vi "G#Debugger_ProxyCall.vi"(0 "Method":i32, 1 "ObjectID":u32, 2 "ObjectAttributes (T)":bool=TRUE, 4 "Text":string, 5 "error in (no error)":errorcluster) -> (15 "Attributes":variant[](array[variant]), 16 "AllObjects":T1(array[cluster]), 17 "ObjectIDs":u32[](array[numeric]), 18 "ValidObject":bool, 19 "error out":errorcluster)   [LabVIEW 2020, in "G#Debugger.lvlib"]
uses:
  <vilib>/addons/_AddQ/G#Debugger/G#Debugger.lvlib
  <vilib>/addons/_AddQ/G#Object/G#Object.lvclass
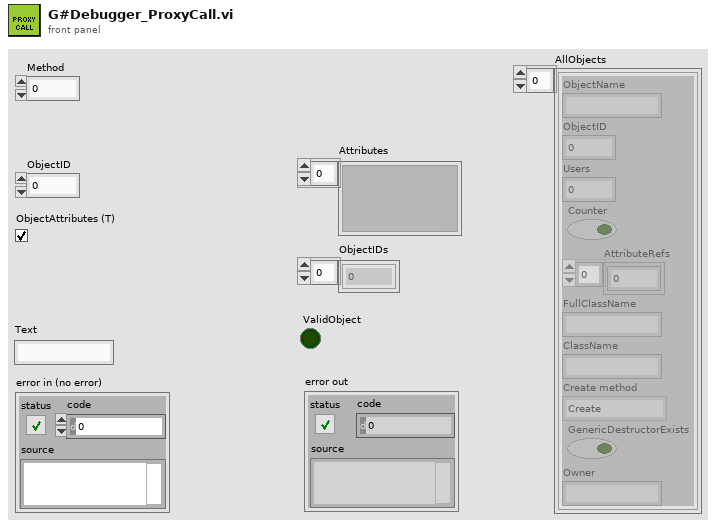
[diagram p1: front panel]
types:
  T1 = cluster{"ObjectName":string, "ObjectID":u32, "Users":i32, "Counter":bool, "AttributeRefs":u32[], "FullClassName":string, "ClassName":string, "Create method":enum16{"Create", "Create or look up existing", "Look up existing"}, "GenericDestructorExists":bool, "Owner":string}[]
  T2 = typedef "G#Object.lvclass/G#Object_ObjectInfoType.ctl" = cluster{"ObjectName":string, "ObjectID":u32, "Users":i32, "Counter":bool, "AttributeRefs":u32[], "FullClassName":string, "ClassName":string, "CreateMethod":T3, "GenericDestructorExists":bool, "Owner":string}
  T3 = typedef "G#Object.lvclass/G#Object_CreateMethod.ctl" = enum16{"Create", "Create or look up existing", "Look up existing"}
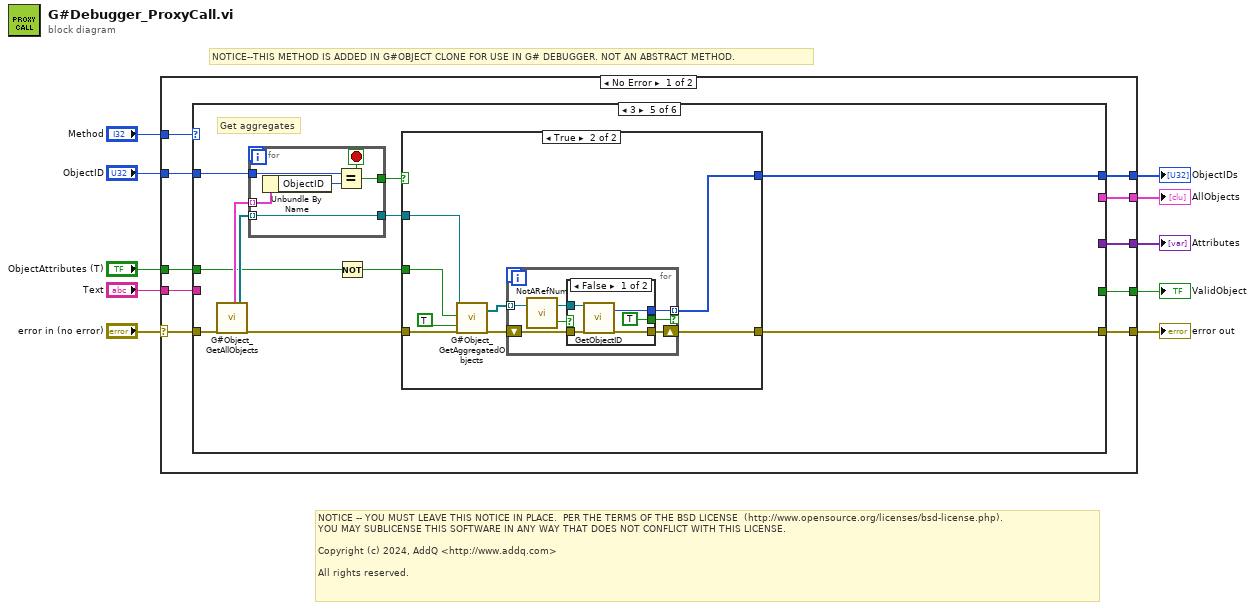
[diagram p0: block diagram]
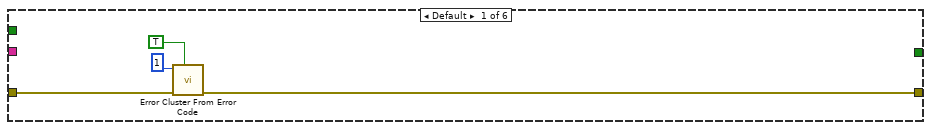
[diagram p2: hidden frame]
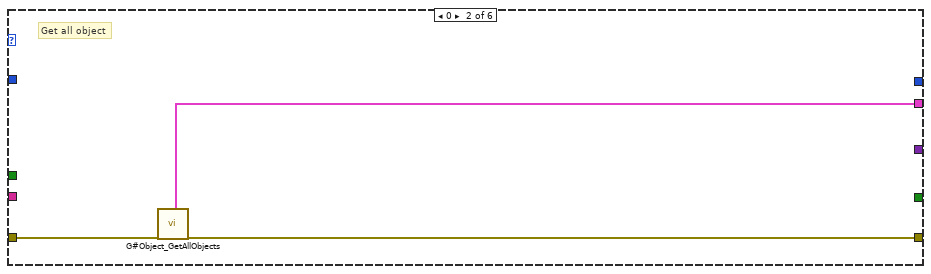
[diagram p3: hidden frame]
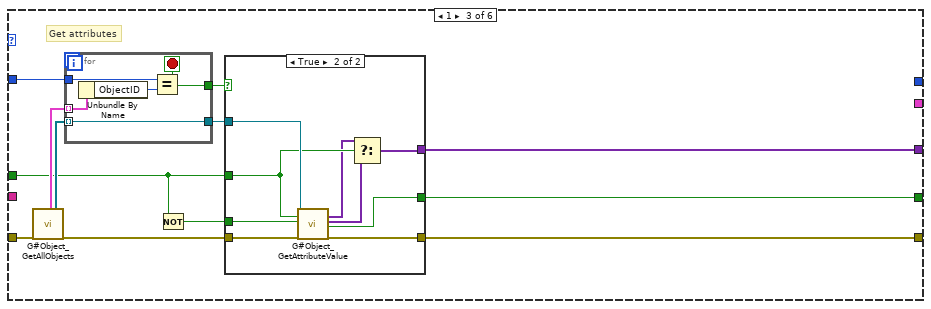
[diagram p4: hidden frame]
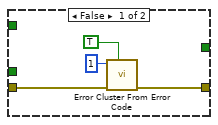
[diagram p5: hidden frame]
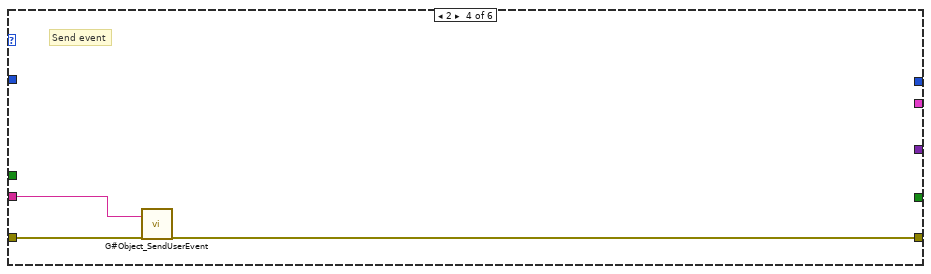
[diagram p6: hidden frame]
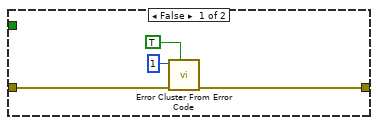
[diagram p7: hidden frame]
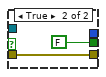
[diagram p8: hidden frame]
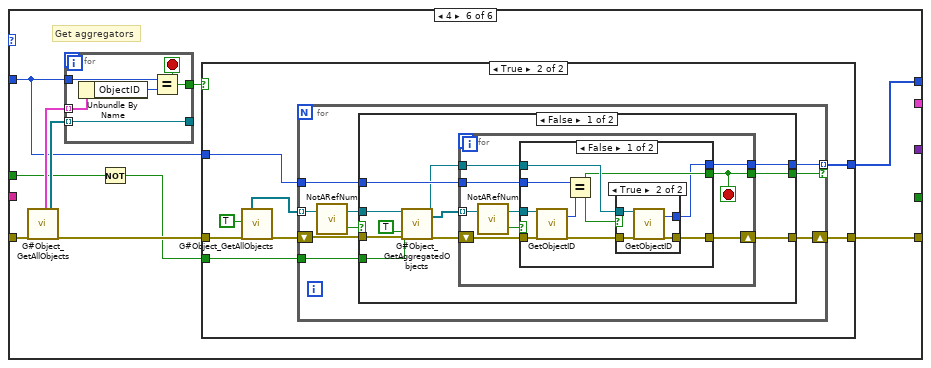
[diagram p9: hidden frame]
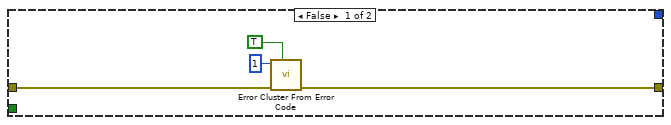
[diagram p10: hidden frame]
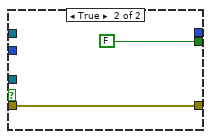
[diagram p12: hidden frame]
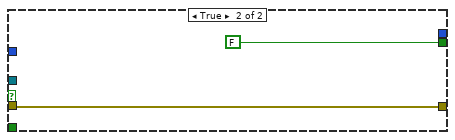
[diagram p13: hidden frame]
diagram:
  # "NOTICE--THIS METHOD IS ADDED IN G#OBJECT CLONE FOR USE IN G# DEBUGGER. NOT AN ABSTRACT METHOD."
  # "NOTICE -- YOU MUST LEAVE THIS NOTICE IN PLACE.  PER THE TERMS OF THE BSD LICENSE  (http://www.opensource.org/licenses/bsd-license.php).\nYOU MAY SUBLICENSE THIS SOFTWARE IN ANY WAY THAT DOES NOT CONFLICT WITH THIS LICENSE.\n\nCopyright (c) 2024, AddQ <http://www.addq.com>\n\nAll rights reserved."
  n1 = case shown="No Error" "error in (no error)" {
    selector: "error in (no error)" -> [w17 w177]
    tunnel: "ObjectID" -> [w20 _]
    tunnel: "ObjectAttributes (T)" -> [w16 _]
    tunnel: [w19 w177] -> w8
    tunnel: [w15 _] -> w7
    tunnel: [w18 _] -> w6
    tunnel: "Method" -> [w14 _]
    tunnel: [w13 _] -> w3
    tunnel: "Text" -> [w12 _]
    tunnel: [w11 _] -> w1
    frame No Error {
      n2 = case shown="3" w14 {
        tunnel: w20 -> [_ _ w38 _ w70 w106]
        tunnel: [w21 w26 w34 w59 w62 w103] -> w19
        tunnel: [_ _ w33 _ _ _] -> w18
        tunnel: w17 -> [w23 w27 w32 w60 w68 w110]
        tunnel: w16 -> [_ _ w30 _ w67 w109]
        tunnel: [_ _ w29 _ _ _] -> w15
        tunnel: [_ w25 _ _ _ _] -> w13
        tunnel: w12 -> [_ _ _ w58 _ _]
        tunnel: [_ _ _ _ w63 w104] -> w11
        frame Default {
          n3 = call <vilib>:"Error Cluster From Error Code.vi"("show call chain? (False)"=TRUE, "error in (no error)"=w23, "error code (0)"=1) -> ("error out"=w21:errorcluster)  [unwired: 6 in]
        }
        frame 0 {
          # "Get all object"
          n4 = call <vilib>:"G#Object_GetAllObjects.vi"("error in (no error)"=w27) -> ("all objects"=w25:T2[], "error out"=w26:errorcluster)  [unwired: 15 in, 2 out]
        }
        frame 1 {
          # "Get attributes"
          n5 = call <vilib>:"G#Object_GetAllObjects.vi"("error in (no error)"=w32) -> ("all objects"=w39:T2[], "all refs"=w37:refnum<class "G#Object.lvclass">[], "error out"=w35:errorcluster)  [unwired: 15 in, 1 out]
          n6 = for {
            tunnel: w39 -> [w55] mode=indexing
            tunnel: w38 -> [w57]
            tunnel: w37 -> [w54] mode=indexing
            tunnel: [w54] -> w36
            tunnel: [w53] -> w28
            stop <- w53 stop-if-true
            n7 = Unbundle By Name(w55) -> ("ObjectID"=w56:u32)
            n8 = Equal?(x=w57, y=w56) -> (x = y?=w53:bool)
          }
          n9 = Not(x=w30) -> (.not. x?=w31:bool)
          n10 = case shown="True" w28 {
            tunnel: w36 -> [_ w52]
            tunnel: w35 -> [w41 w51]
            tunnel: [w40 w50] -> w34
            tunnel: [_ w49] -> w33
            tunnel: w31 -> [_ w48]
            tunnel: w30 -> [_ w47]
            tunnel: [_ w44] -> w29
            frame False {
              n11 = call <vilib>:"Error Cluster From Error Code.vi"("show call chain? (False)"=TRUE, "error in (no error)"=w41, "error code (0)"=1) -> ("error out"=w40:errorcluster)  [unwired: 6 in]
            }
            frame True {
              n12 = call <vilib>:"G#Object_GetAttributeValue.vi"("reference in"=w52, "object attributes (T)"=w47, "class attributes (F)"=w48, "error in (no error)"=w51) -> ("attributes"=w45:variant[], "class attributes"=w46:variant[], "valid object"=w49:bool, "error out"=w50:errorcluster)  [unwired: 11 in, 1 out]
              n13 = Select(t=w45, s=w47, f=w46) -> (s? t:f=w44:variant[])
            }
          }
        }
        frame 2 {
          # "Send event"
          n14 = call <vilib>:"G#Object_SendUserEvent.vi"("text"=w58, "error in (no error)"=w60) -> ("error out"=w59:errorcluster)  [unwired: 16 in, 1 out]
        }
        frame 3 {
          # "Get aggregates"
          n15 = call <vilib>:"G#Object_GetAllObjects.vi"("error in (no error)"=w68) -> ("all objects"=w71:T2[], "all refs"=w69:refnum<class "G#Object.lvclass">[], "error out"=w64:errorcluster)  [unwired: 15 in, 1 out]
          n16 = for {
            tunnel: w71 -> [w100] mode=indexing
            tunnel: w70 -> [w102]
            tunnel: w69 -> [w99] mode=indexing
            tunnel: [w99] -> w66
            tunnel: [w98] -> w61
            stop <- w98 stop-if-true
            n17 = Unbundle By Name(w100) -> ("ObjectID"=w101:u32)
            n18 = Equal?(x=w102, y=w101) -> (x = y?=w98:bool)
          }
          n19 = Not(x=w67) -> (.not. x?=w65:bool)
          n20 = case shown="True" w61 {
            tunnel: w66 -> [_ w81]
            tunnel: w65 -> [_ w80]
            tunnel: w64 -> [w73 w79]
            tunnel: [_ w78] -> w63
            tunnel: [w72 w77] -> w62
            frame False {
              n21 = call <vilib>:"Error Cluster From Error Code.vi"("show call chain? (False)"=TRUE, "error in (no error)"=w73, "error code (0)"=1) -> ("error out"=w72:errorcluster)  [unwired: 6 in]
            }
            frame True {
              n22 = call <vilib>:"G#Object_GetAggregatedObjects.vi"("reference in"=w81, "class attributes (F)"=w80, "remove duplicates (F)"=TRUE, "error in (no error)"=w79) -> ("aggregated objects"=w83:refnum<class "G#Object.lvclass">[], "error out"=w82:errorcluster)  [unwired: 12 in, 2 out]
              n23 = for {
                tunnel: w83 -> [w87] mode=indexing
                shift-right: [w88] -> w77
                shift-left: w82 -> [w90]
                tunnel: [w89] -> w78 mode=indexing if=w84
                n24 = call-dynamic "NotARefNum.vi"("reference in"=w87) -> ("not a refnum?"=w86:bool, "reference out"=w85:refnum<class "G#Object.lvclass">)  [unwired: 1 in]
                n25 = case shown="False" w86 {
                  tunnel: w85 -> [w95 _]
                  tunnel: w90 -> [w94 w97]
                  tunnel: [w92 _] -> w89
                  tunnel: [w93 w97] -> w88
                  tunnel: [TRUE FALSE] -> w84
                  frame False {
                    n26 = call-dynamic "GetObjectID.vi"("reference in"=w95, "error in (no error)"=w94) -> ("object ID"=w92:u32, "error out"=w93:errorcluster)  [unwired: 15 in, 1 out]
                  }
                  frame True {
                  }
                }
              }
            }
          }
        }
        frame 4 {
          # "Get aggregators"
          n27 = call <vilib>:"G#Object_GetAllObjects.vi"("error in (no error)"=w110) -> ("all objects"=w112:T2[], "all refs"=w111:refnum<class "G#Object.lvclass">[], "error out"=w107:errorcluster)  [unwired: 15 in, 1 out]
          n28 = for {
            tunnel: w112 -> [w174] mode=indexing
            tunnel: w106 -> [w176]
            tunnel: w111 -> [w173] mode=indexing
            tunnel: [w173] -> _
            tunnel: [w172] -> w108
            stop <- w172 stop-if-true
            n29 = Unbundle By Name(w174) -> ("ObjectID"=w175:u32)
            n30 = Equal?(x=w176, y=w175) -> (x = y?=w172:bool)
          }
          n31 = Not(x=w109) -> (.not. x?=w105:bool)
          n32 = case shown="True" w108 {
            tunnel: w107 -> [w114 w119]
            tunnel: w105 -> [_ w124]
            tunnel: w106 -> [_ w121]
            tunnel: [w113 w117] -> w103
            tunnel: [_ w120] -> w104
            frame False {
              n33 = call <vilib>:"Error Cluster From Error Code.vi"("show call chain? (False)"=TRUE, "error in (no error)"=w114, "error code (0)"=1) -> ("error out"=w113:errorcluster)  [unwired: 6 in]
            }
            frame True {
              n34 = call <vilib>:"G#Object_GetAllObjects.vi"("only refs (F)"=TRUE, "error in (no error)"=w119) -> ("all refs"=w123:refnum<class "G#Object.lvclass">[], "error out"=w118:errorcluster)  [unwired: 14 in, 2 out]
              n35 = for {
                tunnel: w124 -> [w132]
                shift-right: [w131] -> w117
                shift-left: w118 -> [w133]
                tunnel: w123 -> [w130] mode=indexing
                tunnel: [w126] -> w120 mode=indexing if=w127
                tunnel: w121 -> [w128]
                n36 = call-dynamic "NotARefNum.vi"("reference in"=w130) -> ("not a refnum?"=w129:bool, "reference out"=w125:refnum<class "G#Object.lvclass">)  [unwired: 1 in]
                n37 = case shown="False" w129 {
                  tunnel: w133 -> [w144 w171]
                  tunnel: w132 -> [w143 _]
                  tunnel: [w135 w171] -> w131
                  tunnel: w125 -> [w142 _]
                  tunnel: w128 -> [w139 _]
                  tunnel: [w138 FALSE] -> w127
                  tunnel: [w136 _] -> w126
                  frame False {
                    n38 = call <vilib>:"G#Object_GetAggregatedObjects.vi"("reference in"=w142, "class attributes (F)"=w143, "remove duplicates (F)"=TRUE ("remove duplicates"), "error in (no error)"=w144) -> ("reference out"=w137:refnum<class "G#Object.lvclass">, "aggregated objects"=w141:refnum<class "G#Object.lvclass">[], "error out"=w140:errorcluster)  [unwired: 12 in, 1 out]
                    n39 = for {
                      tunnel: w141 -> [w153] mode=indexing
                      shift-right: [w145] -> w135
                      shift-left: w140 -> [w150]
                      tunnel: w139 -> [w149]
                      tunnel: [w148] -> w138
                      tunnel: w137 -> [w147]
                      tunnel: [w146] -> w136
                      stop <- w148 stop-if-true
                      n40 = call-dynamic "NotARefNum.vi"("reference in"=w153) -> ("not a refnum?"=w152:bool, "reference out"=w151:refnum<class "G#Object.lvclass">)  [unwired: 1 in]
                      n41 = case shown="False" w152 {
                        tunnel: w151 -> [w162 _]
                        tunnel: w150 -> [w161 w168]
                        tunnel: [w157 FALSE] -> w148
                        tunnel: w149 -> [w159 _]
                        tunnel: w147 -> [w158 _]
                        tunnel: [w155 _] -> w146
                        tunnel: [w154 w168] -> w145
                        frame False {
                          n42 = call-dynamic "GetObjectID.vi"("reference in"=w162, "error in (no error)"=w161) -> ("object ID"=w160:u32, "error out"=w156:errorcluster)  [unwired: 15 in, 1 out]
                          n43 = Equal?(x=w159, y=w160) -> (x = y?=w157:bool)
                          n44 = case shown="True" w157 {
                            tunnel: w158 -> [_ w167]
                            tunnel: w156 -> [w163 w166]
                            tunnel: [_ w165] -> w155
                            tunnel: [w163 w164] -> w154
                            frame False {
                            }
                            frame True {
                              n45 = call-dynamic "GetObjectID.vi"("reference in"=w167, "error in (no error)"=w166) -> ("object ID"=w165:u32, "error out"=w164:errorcluster)  [unwired: 15 in, 1 out]
                            }
                          }
                        }
                        frame True {
                        }
                      }
                    }
                  }
                  frame True {
                  }
                }
              }
            }
          }
        }
      }
    }
    frame Error {
    }
  }
  "error out" <- w8
  "Attributes" <- w7
  "ValidObject" <- w6
  "AllObjects" <- w3
  "ObjectIDs" <- w1
